vi "ma_align N waveforms (global interval).vi"(0 "waveforms in":waveform(dbl)[](array[waveform]), 11 "error in":errorcluster, 12 "timestamp difference control":dbl=10.0 format="%.2f") -> (4 "waveforms out":waveform(dbl)[](array[waveform]), 15 "error out":errorcluster)   [LabVIEW 2020, in "NI_MAPro.lvlib"]
uses:
  NI_MAPro.lvlib
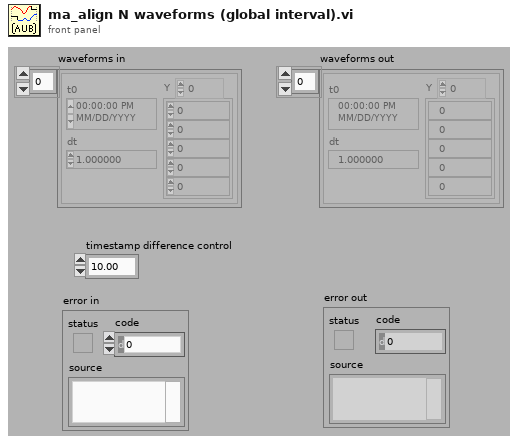
[diagram p1: front panel]
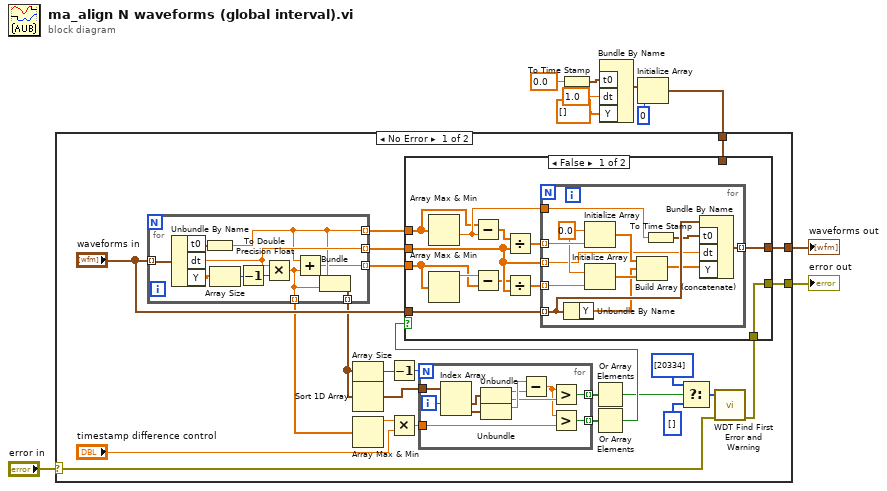
[diagram p0: block diagram]
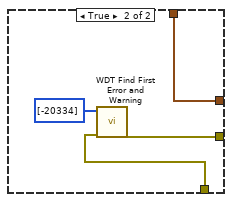
[diagram p2: hidden frame]
diagram:
  n1 = To Time Stamp(1:0.0 ("t0")) -> (0:w1:timestamp)
  n2 = Bundle By Name("t0"=w1, "dt"=1.0, "Y"=dbl[] []) -> (w6:waveform(dbl))  [unwired: 1 in]
  n3 = Initialize Array(w6, 0 ("dimension size")) -> (w2:waveform(dbl)[])
  n4 = case shown="No Error" "error in" {
    selector: "error in" -> [w33 w85]
    tunnel: [w34 w85] -> w10
    tunnel: [w32 w84] -> w8
    tunnel: w2 -> [w30 w84]
    frame No Error {
      n5 = for {
        tunnel: "waveforms in" -> [w83] mode=indexing
        tunnel: [w75] -> w25 mode=indexing
        tunnel: [w78] -> w26 mode=indexing
        tunnel: [w79] -> w29 mode=indexing
        tunnel: [w77] -> w28 mode=indexing
        tunnel: [w76] -> w20 mode=indexing
        n6 = Unbundle By Name(w83) -> ("t0"=w74:timestamp, "dt"=w79:dbl, "Y"=w80:dbl[])
        n7 = To Double Precision Float(number=w74) -> (double precision float=w78:dbl)
        n8 = Array Size(array=w80) -> (size(s)=w82:i32)
        n9 = Decrement(x=w82) -> (x-1=w81:i32)
        n10 = Multiply(x=w79, y=w81) -> (x*y=w76:dbl)
        n11 = Add(x=w78, y=w76) -> (x+y=w75:dbl)
        n12 = Bundle(w78, w76) -> (w77:cluster{dbl, dbl})  [unwired: 1 in]
      }
      n13 = Array Size(array=w28) -> (size(s)=w27:i32)
      n14 = Sort 1D Array(array=w28) -> (sorted array=w23:cluster{dbl, dbl}[])
      n15 = Array Max & Min(array=w20) -> (max value=w19:dbl)  [unwired: 3 out]
      n16 = Decrement(x=w27) -> (x-1=w24:i32)
      n17 = Multiply(x=w19, y="timestamp difference control") -> (x*y=w17:dbl)
      n18 = for {
        N: w24 -> [_]
        tunnel: w23 -> [w73]
        tunnel: [w69] -> w16 mode=indexing
        tunnel: [w65] -> w22 mode=indexing
        tunnel: w17 -> [w64]
        i -> [w72]
        n19 = Index Array(array=w73, index #1=w72) -> (element #1=w71:cluster{dbl, dbl}, element #2=w70:cluster{dbl, dbl})  [unwired: 1 in]
        n20 = Unbundle(w71) -> (w67:dbl, w66:dbl)
        n21 = Unbundle(w70) -> (w68:dbl)  [unwired: 1 out]
        n22 = Subtract(x=w68, y=w67) -> (x-y=w63:dbl)
        n23 = Greater?(x=w63, y=w66) -> (0:w69:bool)
        n24 = Greater?(x=w63, y=w64) -> (0:w65:bool)
      }
      n25 = Or Array Elements(Boolean array=w16) -> (logical OR=w12:bool)
      n26 = Or Array Elements(Boolean array=w22) -> (logical OR=w21:bool)
      n27 = Select(t=i32[] [20334] ("Error Codes"), s=w12, f=i32[] [] ("Error Codes")) -> (s? t:f=w15:i32[])
      n28 = call "WDT Find First Error and Warning.vi"("error in (no error)"=w33, "Error Codes"=w15) -> ("error out"=w11:errorcluster)  [unwired: 4 in, 1 out]
      n29 = case shown="False" w21 {
        tunnel: w29 -> [w46 _]
        tunnel: [w40 w62] -> w32
        tunnel: "waveforms in" -> [w39 _]
        tunnel: w26 -> [w37 _]
        tunnel: w25 -> [w36 _]
        tunnel: w30 -> [_ w62]
        tunnel: w11 -> [w35 w60]
        tunnel: [w35 w61] -> w34
        frame False {
          n30 = Array Max & Min(array=w37) -> (min value=w38:dbl)  [unwired: 3 out]
          n31 = Array Max & Min(array=w36) -> (max value=w41:dbl)  [unwired: 3 out]
          n32 = Subtract(x=w37, y=w38) -> (x-y=w42:dbl[])
          n33 = Subtract(x=w41, y=w36) -> (x-y=w43:dbl[])
          n34 = Divide(x=w42, y=w46) -> (x/y=w44:dbl[])
          n35 = Divide(x=w43, y=w46) -> (x/y=w45:dbl[])
          n36 = for {
            tunnel: w39 -> [w58] mode=indexing
            tunnel: w44 -> [w57] mode=indexing
            tunnel: w45 -> [w56] mode=indexing
            tunnel: w46 -> [w50] mode=indexing
            tunnel: w38 -> [w49]
            tunnel: [w48] -> w40 mode=indexing
            w55 = 0.0 ("element")
            n37 = Unbundle By Name(w58) -> ("Y"=w52:dbl[])
            n38 = Initialize Array(w55, w57) -> (w54:dbl[])
            n39 = Initialize Array(w55, w56) -> (w53:dbl[])
            n40 = Build Array (concatenate)(w54, w52, w53) -> (w51:dbl[])
            n41 = To Time Stamp(1:w49) -> (0:w47:timestamp)
            n42 = Bundle By Name(cluster=w58, "t0"=w47, "dt"=w50, "Y"=w51) -> (w48:waveform(dbl))
          }
        }
        frame True {
          n43 = call "WDT Find First Error and Warning.vi"("error in (no error)"=w60, "Error Codes"=i32[] [-20334]) -> ("error out"=w61:errorcluster)  [unwired: 4 in, 1 out]
        }
      }
    }
    frame Error {
    }
  }
  "error out" <- w10
  "waveforms out" <- w8
